vi "Get DAQ Settings.vi"(8 "error in (no error)":errorcluster, 10 "Physical Chan Array":i32[](array[numeric]), 11 "Device Ref in":T1 format="%.0x") -> (0 "error out":errorcluster, 2 "DAQ Config Data":T2, 3 "Device Ref Out":T1 format="%.0x")   [LabVIEW 2023, in "Waveform Analog Output Engine.lvlib"]
doc: "Reads all of the DAQ configuration properties from the custom device"
uses:
  Waveform Analog Output Engine.lvlib
  <vilib>/NI VeriStand/Custom Device API/Custom Device Item Ref.ctl
  DAQ Config Data.ctl
  Shared/Constants.vi
  <vilib>/NI VeriStand/Custom Device API/Get Item Property (String).vi
  <vilib>/NI VeriStand/Custom Device API/Get Item Property (Double).vi
  <vilib>/NI VeriStand/Custom Device API/Custom Device API.lvlib
  Shared/Waveform Analog Output Shared.lvlib
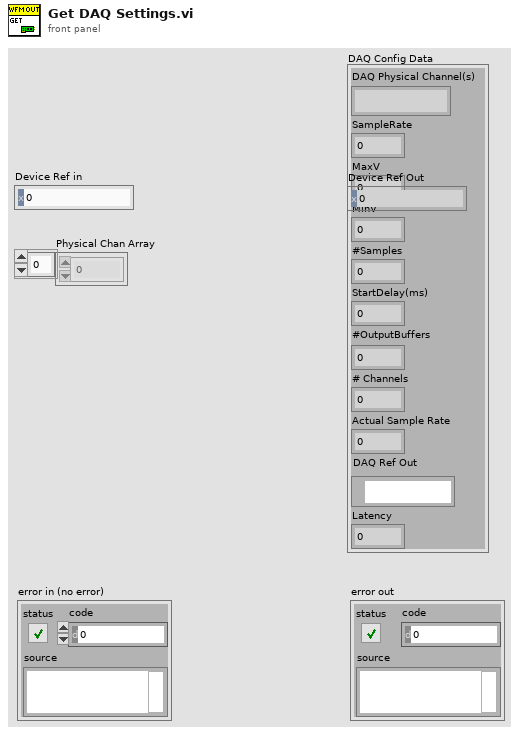
[diagram p1: front panel]
types:
  T1 = typedef "Custom Device API.lvlib/Custom Device Item Ref.ctl" = u64
  T2 = typedef "Waveform Analog Output Engine.lvlib/DAQ Config Data.ctl" = cluster{"DAQ Physical Channel(s)":string, "SampleRate":dbl, "MaxV":dbl, "MinV":dbl, "#Samples":dbl, "StartDelay(ms)":dbl, "#OutputBuffers":dbl, "# Channels":i32, "Actual Sample Rate":dbl, "DAQ Ref Out":refnum<k21>, "Latency":dbl}
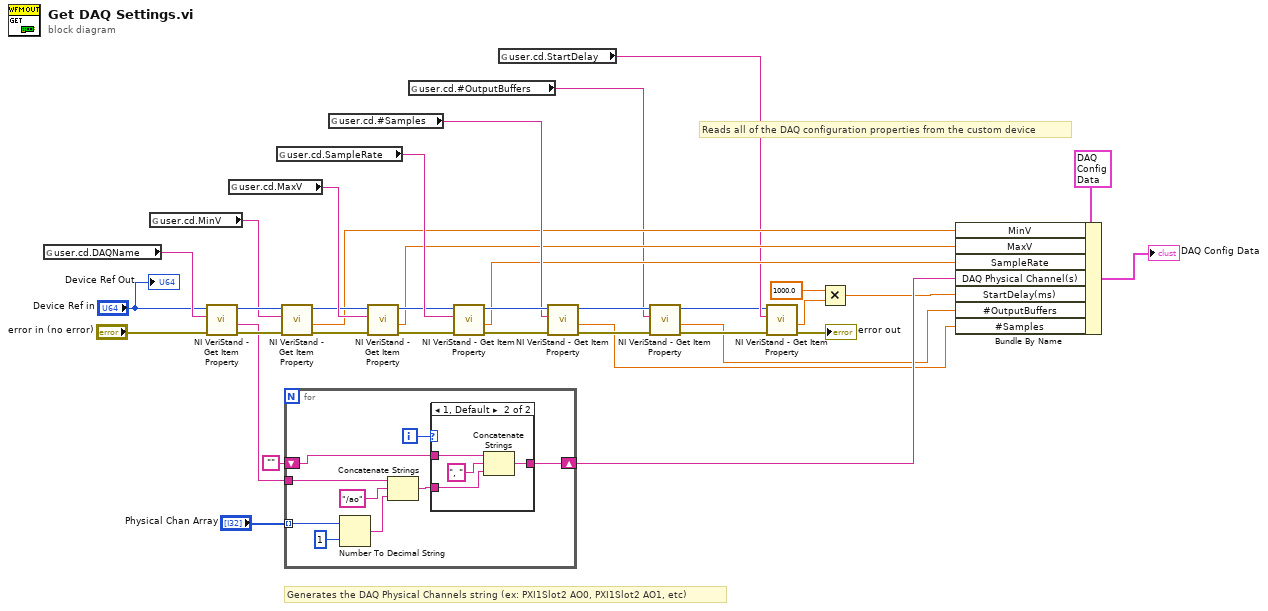
[diagram p0: block diagram]
diagram:
  # "Generates the DAQ Physical Channels string (ex: PXI1Slot2 AO0, PXI1Slot2 AO1, etc)"
  # "Reads all of the DAQ configuration properties from the custom device"
  n1 = global read "Constants.vi" "user.cd.DAQName"() -> (w34:string)
  n2 = global read "Constants.vi" "user.cd.MinV"() -> (w25:string)
  n3 = call-poly <vilib>:"NI VeriStand - Get Item Property.vi"("error in (no error)"="error in (no error)", "Property Name"=w34, "Item Ref in"="Device Ref in") -> ("error out"=w31:errorcluster, "Value"=w22:string, "Item Ref out"=w30:T1)  [unwired: 5 in, 1 out]
  n4 = global read "Constants.vi" "user.cd.MaxV"() -> (w26:string)
  n5 = global read "Constants.vi" "user.cd.SampleRate"() -> (w29:string)
  n6 = call-poly <vilib>:"NI VeriStand - Get Item Property.vi"("error in (no error)"=w31, "Property Name"=w25, "Item Ref in"=w30) -> ("error out"=w24:errorcluster, "Value"=w17:dbl, "Item Ref out"=w23:T1)  [unwired: 5 in, 1 out]
  n7 = for {
    tunnel: w22 -> [w43]
    shift-right: [w38] -> w14
    shift-left: "" -> [w37]
    tunnel: "Physical Chan Array" -> [w42] mode=indexing
    i -> [w45]
    n8 = Number To Decimal String(number=w42, width (-)=i16 1) -> (decimal integer string=w40:string)
    n9 = Concatenate Strings(w43, "/ao" ("string"), w40) -> (w39:string)
    n10 = case shown="1, Default" w45 {
      tunnel: w39 -> [w46 w49]
      tunnel: [w46 w48] -> w38
      tunnel: w37 -> [_ w47]
      frame 0 {
      }
      frame 1, Default {
        n11 = Concatenate Strings(w47, ", " ("string"), w49) -> (w48:string)
      }
    }
  }
  n12 = global read "Constants.vi" "user.cd.#Samples"() -> (w19:string)
  n13 = call-poly <vilib>:"NI VeriStand - Get Item Property.vi"("error in (no error)"=w24, "Property Name"=w26, "Item Ref in"=w23) -> ("error out"=w28:errorcluster, "Value"=w16:dbl, "Item Ref out"=w27:T1)  [unwired: 5 in, 1 out]
  n14 = global read "Constants.vi" "user.cd.#OutputBuffers"() -> (w6:string)
  n15 = call-poly <vilib>:"NI VeriStand - Get Item Property.vi"("error in (no error)"=w28, "Property Name"=w29, "Item Ref in"=w27) -> ("error out"=w21:errorcluster, "Value"=w15:dbl, "Item Ref out"=w20:T1)  [unwired: 5 in, 1 out]
  n16 = global read "Constants.vi" "user.cd.StartDelay"() -> (w11:string)
  n17 = call-poly <vilib>:"NI VeriStand - Get Item Property.vi"("error in (no error)"=w21, "Property Name"=w19, "Item Ref in"=w20) -> ("error out"=w7:errorcluster, "Value"=w1:dbl, "Item Ref out"=w8:T1)  [unwired: 5 in, 1 out]
  n18 = call-poly <vilib>:"NI VeriStand - Get Item Property.vi"("error in (no error)"=w7, "Property Name"=w6, "Item Ref in"=w8) -> ("error out"=w4:errorcluster, "Value"=w2:dbl, "Item Ref out"=w5:T1)  [unwired: 5 in, 1 out]
  n19 = call-poly <vilib>:"NI VeriStand - Get Item Property.vi"("error in (no error)"=w4, "Property Name"=w11, "Item Ref in"=w5) -> ("error out"=→"error out":errorcluster, "Value"=w10:dbl)  [unwired: 5 in, 2 out]
  n20 = Multiply(x=1000.0, y=w10) -> (x*y=w3:dbl)
  n21 = Bundle By Name(cluster=T2 {"DAQ Physical Channel(s)"="", "SampleRate"=0.0, "MaxV"=0.0, "MinV"=0.0, "#Samples"=0.0, "StartDelay(ms)"=0.0, "#OutputBuffers"=0.0, "# Channels"=0, "Actual Sample Rate"=0.0, "DAQ Ref Out"="", "Latency"=0.0} ("DAQ Config Data"), "MinV"=w17, "MaxV"=w16, "SampleRate"=w15, "DAQ Physical Channel(s)"=w14, "StartDelay(ms)"=w3, "#OutputBuffers"=w2, "#Samples"=w1) -> (→"DAQ Config Data":T2)
  "Device Ref Out" <- "Device Ref in"
